vi "meta_unflattenBlockHeader.vi"(11 "block header data":u8[](array[numeric])) -> (3 "block out":T1={"Version"=10, "Type"=enum."File", "Length"=0, "Data"=""})   [LabVIEW 2020, in "NI_ExcelFile.lvlib"]
uses:
  <vilib>/express/express shared/NI_ExcelFile/NI_ExcelFile.lvlib
  <vilib>/express/express shared/NI_ExcelFile/Ctrls/meta_Block.ctl
  <vilib>/express/express shared/NI_ExcelFile/Ctrls/meta_BlockType.ctl
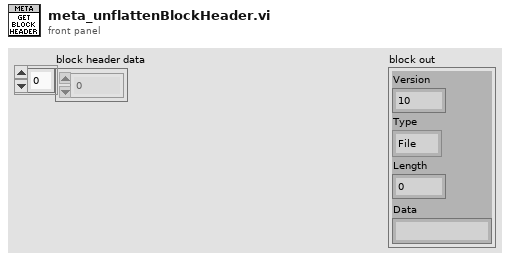
[diagram p1: front panel]
types:
  T1 = typedef "NI_ExcelFile.lvlib/meta_Block.ctl" = cluster{"Version":u16, "Type":T2, "Length":i32, "Data":string}
  T2 = typedef "NI_ExcelFile.lvlib/meta_BlockType.ctl" = enum16{"NITag", "File", "Column"}
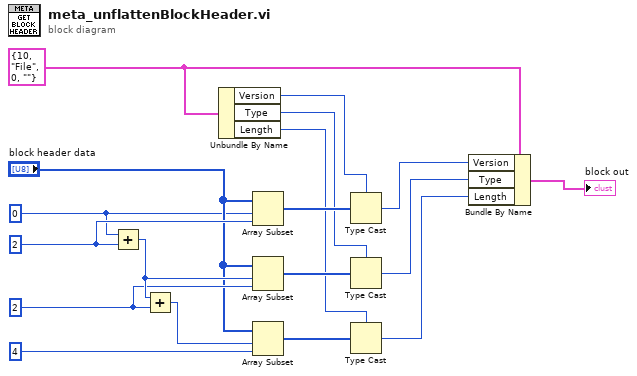
[diagram p0: block diagram]
diagram:
  w7 = T1 {"Version"=10, "Type"=enum."File", "Length"=0, "Data"=""} ("Block")
  w9 = 2 ("length")
  w8 = 2 ("length")
  w1 = 0 ("index")
  n1 = Add(x=w1, y=w8) -> (x+y=w10:i32)
  n2 = Add(x=w10, y=w9) -> (x+y=w3:i32)
  n3 = Unbundle By Name(w7) -> ("Version"=w13:u16, "Type"=w12:T2, "Length"=w11:i32)
  n4 = Array Subset(array="block header data", index=w1, length=w8) -> (w18:u8[])
  n5 = Array Subset(array="block header data", index=w10, length=w9) -> (w16:u8[])
  n6 = Array Subset(array="block header data", index=w3, length=4) -> (w15:u8[])
  n7 = Type Cast(type=w13, x=w18) -> (*(type *) &x=w17:u16)
  n8 = Type Cast(type=w12, x=w16) -> (*(type *) &x=w14:T2)
  n9 = Type Cast(type=w11, x=w15) -> (*(type *) &x=w4:i32)
  n10 = Bundle By Name(cluster=w7, "Version"=w17, "Type"=w14, "Length"=w4) -> (→"block out":T1)
